vi "Convert Number to Fault.vi"(11 "Number":i32) -> (3 "Fault":T1=enum."Motor Stall")   [LabVIEW 2020, in "ChromTech Next Gen Pump.lvlib"]
uses:
  ChromTech Next Gen Pump.lvlib
  Typedefs/Faults.ctl
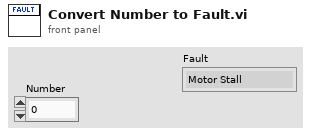
[diagram p1: front panel]
types:
  T1 = typedef "ChromTech Next Gen Pump.lvlib/Faults.ctl" = enum16{"Upper Pressure Fault", "Lower Pressure Fault", "Motor Stall"}
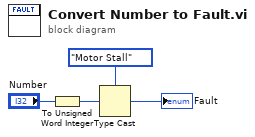
[diagram p0: block diagram]
diagram:
  n1 = To Unsigned Word Integer(number="Number") -> (unsigned 16bit integer=w2:u16)
  n2 = Type Cast(type=Faults."Motor Stall" ("Faults (enum)"), x=w2) -> (*(type *) &x=→"Fault":T1)
